vi "OverlayCrossHatch.vi"(7 "VPI":cluster{"Offset":T1, "Scale":T1}={"Offset"={"X"=0.0, "Y"=0.0}, "Scale"={"X"=1.0, "Y"=1.0}}, 8 "error in (no error)":errorcluster, 9 "Array Size":i32[](array[numeric]), 10 "Cursor Coord":T1, 11 "Vector Image":T2) -> (0 "error out":errorcluster, 2 "Point Location":cluster{dbl, dbl}[](array[cluster]))   [LabVIEW 2022 SP3]
uses:
  <vilib>/Utility/miscctls.llb/LVPointDoubleTypeDef.ctl
  <vilib>/vision/Image Controls.llb/IMAQ Image.ctl
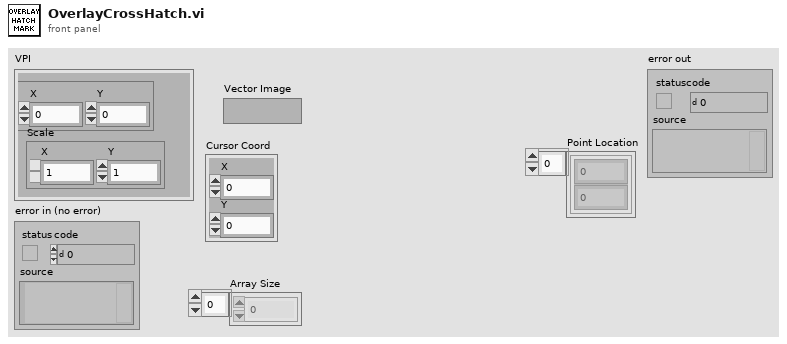
[diagram p1: front panel]
types:
  T1 = typedef "LVPointDoubleTypeDef.ctl" = cluster{"X":dbl, "Y":dbl}
  T2 = typedef "IMAQ Image.ctl" = refnum<image>
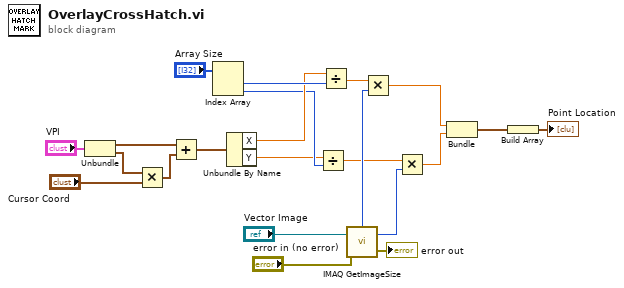
[diagram p0: block diagram]
diagram:
  n1 = Unbundle("VPI") -> ("Offset"=w4:T1, "Scale"=w7:T1)
  n2 = Multiply(x=w7, y="Cursor Coord") -> (x*y=w5:T1)
  n3 = Add(x=w4, y=w5) -> (x+y=w3:T1)
  n4 = Index Array(array="Array Size") -> (element #1=w20:i32, element #2=w18:i32)  [unwired: 2 in]
  n5 = Unbundle By Name(w3) -> ("X"=w19:dbl, "Y"=w17:dbl)
  n6 = Divide(x=w17, y=w18) -> (x/y=w14:dbl)
  n7 = Divide(x=w19, y=w20) -> (x/y=w16:dbl)
  n8 = call "IMAQ GetImageSize"("Image"="Vector Image", "error in (no error)"="error in (no error)") -> ("Y Resolution"=w13:i32, "X Resolution"=w15:i32, "error out"=→"error out":errorcluster)  [unwired: 2 in]
  n9 = Multiply(x=w16, y=w15) -> (x*y=w12:dbl)
  n10 = Multiply(x=w14, y=w13) -> (x*y=w11:dbl)
  n11 = Bundle(w12, w11) -> (w10:cluster{dbl, dbl})  [unwired: 1 in]
  n12 = Build Array(w10) -> (→"Point Location":cluster{dbl, dbl}[])
